vi "exam2.vi"() -> ()   [LabVIEW 2019]
uses:
  <vilib>/myRIO/Instrument Drivers/Onboard IO/DIO/typedefs/DIO Reference.ctl
  <vilib>/myRIO/Common/Instrument Driver Framework/Utilities/typedefs/myRIO Generic Hardware Reference.ctl
  <vilib>/myRIO/Common/Instrument Driver Framework/Utilities/typedefs/Hardware Version Enum.ctl
  <vilib>/myRIO/Common/Instrument Driver Framework/Utilities/typedefs/myRIO v1.0 Reference.ctl
  <vilib>/myRIO/Common/Instrument Driver Framework/Utilities/typedefs/Generic FPGA Reference.ctl
  <vilib>/myRIO/Common/Instrument Driver Framework/myRIO v1.0/DIO/typedefs/DIO Channels List.ctl
  <vilib>/myRIO/Common/Instrument Driver Framework/myRIO v1.0/DIO/typedefs/DIO Channels Enum.ctl
  <vilib>/userDefined/High Color/nirio_resource_hc.ctl
  <vilib>/userDefined/High Color/IMAQdx.ctl
  <vilib>/myRIO/Instrument Drivers/Onboard IO/PWM/typedefs/PWM Reference.ctl
  <vilib>/myRIO/Common/Instrument Driver Framework/myRIO v1.0/PWM/typedefs/PWM Channels Enum.ctl
  <vilib>/myRIO/Instrument Drivers/Onboard IO/PWM/typedefs/PWM Configuration.ctl
  <vilib>/myRIO/Common/Instrument Driver Framework/Utilities/vis/Is FPGA Ref Available.vi
  <vilib>/myRIO/Common/Instrument Driver Framework/myRIO v1.0/DIO/vis/myRIO v1.1 Open DIO.vi
  <vilib>/myRIO/Instrument Drivers/Onboard IO/DIO/vis/Write.vi
  <vilib>/myRIO/Common/Instrument Driver Framework/myRIO v1.0/PWM/vis/myRIO v1.1 Open PWM.vi
  <vilib>/myRIO/Common/Instrument Driver Framework/Utilities/vis/Validate Channels.vi
  <vilib>/myRIO/Common/Instrument Driver Framework/myRIO v1.0/DIO/vis/myRIO v1.0 Reserve DIO.vi
  <vilib>/myRIO/Common/Instrument Driver Framework/myRIO v1.0/PWM/vis/myRIO v1.0 Reserve PWM.vi
  <vilib>/myRIO/Common/Instrument Driver Framework/myRIO v1.0/PWM/vis/myRIO v1.0 Close PWM.vi
  <vilib>/myRIO/Common/Instrument Driver Framework/myRIO v1.0/Resource Manager/vis/myRIO v1.0 Reserve Channel List.vi
  <vilib>/myRIO/Common/Instrument Driver Framework/myRIO v1.0/DIO/vis/myRIO v1.0 Build MUX Configuration DIO.vi
  <vilib>/myRIO/Common/Instrument Driver Framework/myRIO v1.0/PWM/vis/myRIO v1.0 Build MUX Configuration PWM.vi
  <vilib>/myRIO/Common/Instrument Driver Framework/myRIO v1.0/PWM/vis/myRIO v1.0 Unreserve PWM.vi
  <vilib>/myRIO/Common/Instrument Driver Framework/myRIO v1.0/Resource Manager/vis/myRIO v1.0 Reserve Channel.vi
  <vilib>/myRIO/Common/Instrument Driver Framework/myRIO v1.0/Resource Manager/vis/myRIO v1.0 Unreserve Channel.vi
  <vilib>/myRIO/Common/Instrument Driver Framework/myRIO v1.0/Resource Manager/vis/myRIO v1.0 Create Configuration List.vi
  <vilib>/myRIO/Common/Instrument Driver Framework/myRIO v1.0/Resource Manager/vis/myRIO v1.0 Unreserve Channel List.vi
  <vilib>/myRIO/Common/Instrument Driver Framework/myRIO v1.0/Resource Manager/vis/myRIO v1.0 Build Mutex Name.vi
  <vilib>/Utility/VariantDataType/GetNumericInfo.vi
  <vilib>/Utility/error.llb/Error Cluster From Error Code.vi
  <vilib>/myRIO/Common/Instrument Driver Framework/myRIO v1.0/myRIO v1.1 Open.vi
  <vilib>/myRIO/Common/Instrument Driver Framework/Utilities/vis/IO Manager.vi
  <vilib>/myRIO/Common/Instrument Driver Framework/Utilities/vis/Configuration Manager.vi
  <vilib>/myRIO/Common/Instrument Driver Framework/myRIO v1.0/Resource Manager/vis/myRIO v1.0 Configure IO.vi
  <vilib>/myRIO/Common/Instrument Driver Framework/myRIO v1.0/myRIO v1.0 Close.vi
  <vilib>/myRIO/Common/Instrument Driver Framework/myRIO v1.0/PWM/vis/myRIO v1.0 Write PWM.vi
  <vilib>/myRIO/Common/Instrument Driver Framework/myRIO v1.0/PWM/vis/myRIO v1.0 Shutdown PWM.vi
  <vilib>/myRIO/Common/Instrument Driver Framework/myRIO v1.0/DIO/vis/myRIO v1.0 Write DIO.vi
  <vilib>/myRIO/Instrument Drivers/Onboard IO/PWM/vis/myRIO PWM Open.xnode
  <vilib>/myRIO/Express VI/Onboard IO/DO/DO Express VI.xnode
  <vilib>/myRIO/Instrument Drivers/Onboard IO/DIO/vis/myRIO DIO Open.xnode
  <vilib>/myRIO/Instrument Drivers/Onboard IO/PWM/PWM.lvlib
  <vilib>/vision/driver/NI_Vision_Acquisition_Software.lvlib
  <vilib>/myRIO/Instrument Drivers/Onboard IO/DIO/DIO.lvlib
panel:
  out "digital output":bool
  in  "reset":bool
  in  "LED stop":bool
  in  "webcam stop":bool
  out "picture":string
  out "Image":T1(plugin-control)
  in  "stop":bool
  in  "angle":dbl
  out "35«×":bool
  in  "Frequency [Hz]":dbl=1000.0
  out "duty cycle [%]":dbl
  in  "null offset":bool
  out "puls width [ms]":dbl
  out "offset":dbl
  in  "Channel Name":tag
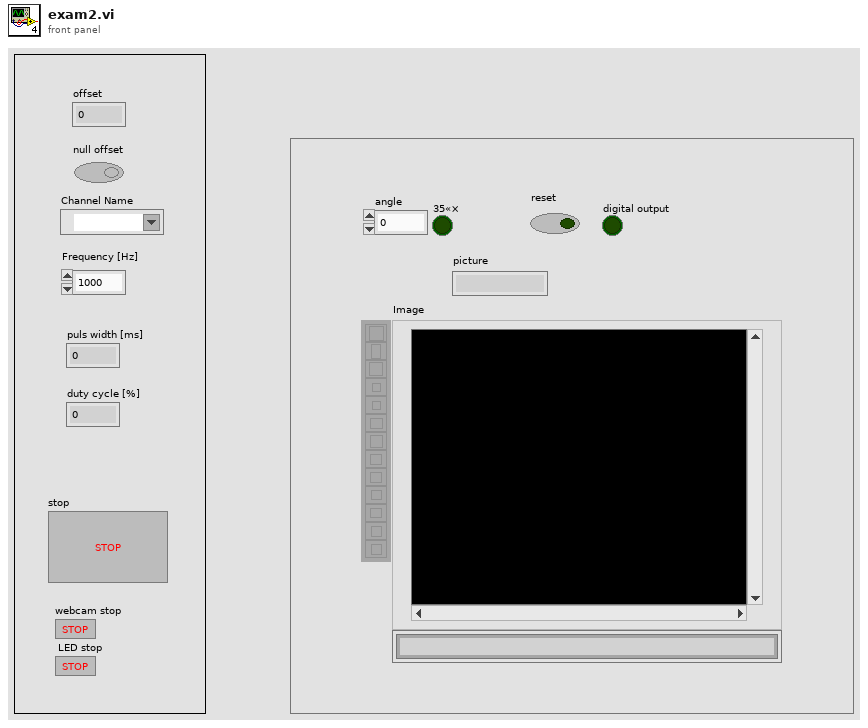
[diagram p1: front panel]
types:
  T1 = typedef "IMAQ Image.ctl" = refnum<image>
  T2 = typedef "PWM.lvlib/PWM Reference.ctl" = cluster{"myRIO Reference":T3, "PWM Channels Enum":T7, "PWM Configuration":T8}
  T3 = typedef "myRIO Generic Hardware Reference.ctl" = cluster{"myRIO Model":T4, "myRIO Hardware Reference":T5}
  T4 = typedef "Hardware Version Enum.ctl" = enum16{"Unknown", "myRIO-1900", "myRIO-1950", "roboRIO", "NI ELVIS RIO CM", "ELVIS III"}
  T5 = typedef "myRIO v1.0 Reference.ctl" = cluster{"Generic FPGA Reference":T6, "Allow multiple opens":bool}
  T6 = typedef "Generic FPGA Reference.ctl" = refnum<k20>
  T7 = typedef "PWM Channels Enum.ctl" = enum16{"Not Connected", "C/PWM0", "C/PWM1", "A/PWM0", "A/PWM1", "A/PWM2", "A/PWM3", "A/PWM4", "A/PWM5", "A/PWM6", "A/PWM7", "A/PWM8", "A/PWM9", "A/PWM10", "A/PWM11", "A/PWM12", "A/PWM13", "A/PWM14", "A/PWM15", "A/PWM16", "A/PWM17", "A/PWM18", "A/PWM19", "B/PWM0", "B/PWM1", "B/PWM2", "B/PWM3", "B/PWM4", "B/PWM5", "B/PWM6", "B/PWM7", "B/PWM8", "B/PWM9", "B/PWM10", "B/PWM11", "B/PWM12", "B/PWM13", "B/PWM14", "B/PWM15", "B/PWM16", "B/PWM17", "B/PWM18", "B/PWM19", "PWM/PWM0", "PWM/PWM1", "PWM/PWM2", "PWM/PWM3", "PWM/PWM4", "PWM/PWM5", "PWM/PWM6", "PWM/PWM7", "PWM/PWM8", "PWM/PWM9"}
  T8 = typedef "PWM.lvlib/PWM Configuration.ctl" = cluster{"Frequency":dbl, "Duty Cycle":dbl}
  T9 = typedef "IMAQdx.ctl" = refnum<k21>
  T10 = typedef "DIO.lvlib/DIO Reference.ctl" = cluster{"myRIO Reference":T3, "DIO Channels List":T11}
  T11 = typedef "DIO Channels List.ctl" = T12[]
  T12 = typedef "DIO Channels Enum.ctl" = enum16{"Not Connected", "C/DIO0", "C/DIO1", "C/DIO2", "C/DIO3", "C/DIO4", "C/DIO5", "C/DIO6", "C/DIO7", "A/DIO0", "A/DIO1", "A/DIO2", "A/DIO3", "A/DIO4", "A/DIO5", "A/DIO6", "A/DIO7", "A/DIO8", "A/DIO9", "A/DIO10", "A/DIO11", "A/DIO12", "A/DIO13", "A/DIO14", "A/DIO15", "A/DIO16", "A/DIO17", "A/DIO18", "A/DIO19", "B/DIO0", "B/DIO1", "B/DIO2", "B/DIO3", "B/DIO4", "B/DIO5", "B/DIO6", "B/DIO7", "B/DIO8", "B/DIO9", "B/DIO10", "B/DIO11", "B/DIO12", "B/DIO13", "B/DIO14", "B/DIO15", "B/DIO16", "B/DIO17", "B/DIO18", "B/DIO19", "LED0", "LED1", "LED2", "LED3", "Button0", "DIO/DIO0", "DIO/DIO1", "DIO/DIO2", "DIO/DIO3", "DIO/DIO4", "DIO/DIO5", "DIO/DIO6", "DIO/DIO7", "DIO/DIO8", "DIO/DIO9", "SPI/CS0", "SPI/CS1", "SPI/CS2", "SPI/CS3", "LED RADIO (Green)", "LED RADIO (Red)", "LED COMM (Green)", "LED COMM (Red)", "LED MODE (Green)", "LED MODE (Red)"}
  T13 = typedef "nirio_resource_hc.ctl" = tag
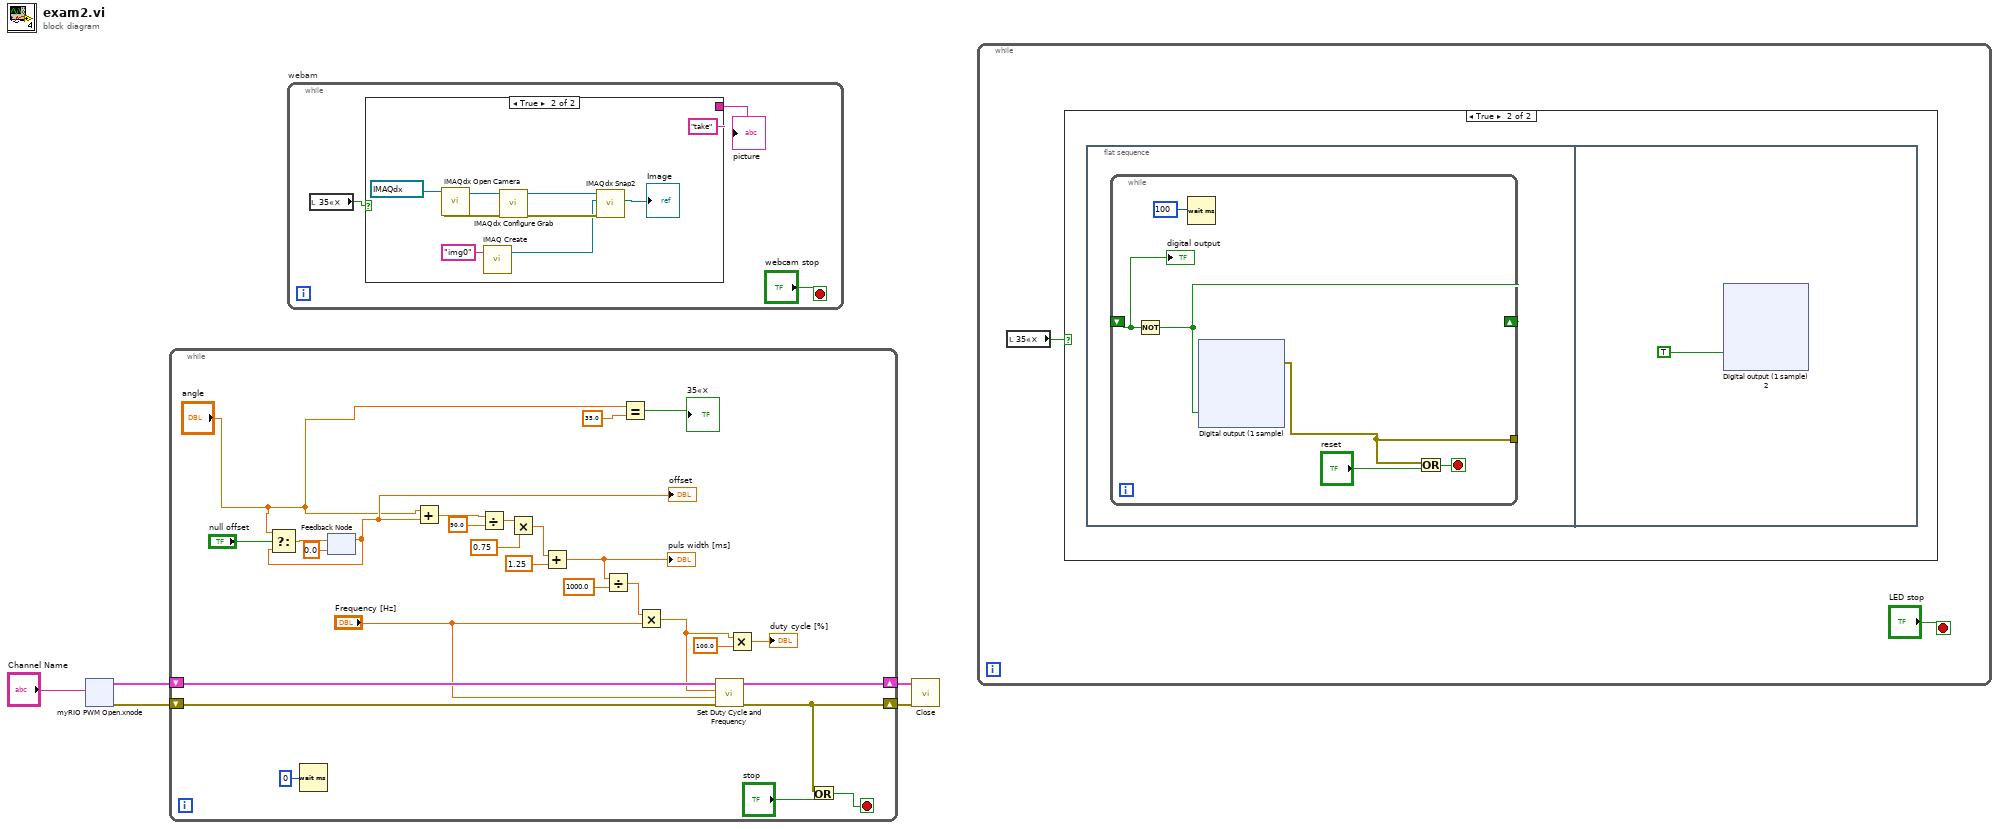
[diagram p0: block diagram]
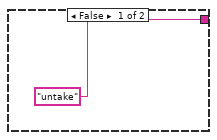
[diagram p3: hidden frame]
diagram:
  n1 = xnode "myRIO PWM Open.xnode"("Channel Name"="Channel Name") -> ("error out"=w4:errorcluster, "PWM Ref Out"=w3:T2)  [unwired: 2 in]
  n2 = while {
    shift-right: [w16] -> w2
    shift-left: w4 -> [w32]
    shift-right: [w30] -> w1
    shift-left: w3 -> [w31]
    stop <- w17 stop-if-true
    n3 = Wait (ms)(milliseconds to wait=u32 0) -> ()  [unwired: 1 out]
    n4 = feedback #1(0.0) -> (w14:dbl)
    "offset" <- w14
    n5 = Select(t="angle", s="null offset", f=w14) -> (s? t:f=w25:dbl)
    n6 = feedback-in #1(w25) -> ()
    n7 = Add(x="angle", y=w14) -> (x+y=w10:dbl)
    n8 = Divide(x=w10, y=90.0) -> (x/y=w13:dbl)
    n9 = Multiply(x=w13, y=0.75) -> (x*y=w12:dbl)
    n10 = Add(x=w12, y=1.25) -> (x+y=w20:dbl)
    "puls width [ms]" <- w20
    n11 = Divide(x=w20, y=1000.0) -> (x/y=w18:dbl)
    n12 = Equal?(x="angle", y=35.0) -> (x = y?=→"35«×":bool)
    n13 = Multiply(x=w18, y="Frequency [Hz]") -> (x*y=w27:dbl)
    n14 = call <vilib>:"Set Duty Cycle and Frequency.vi"("error in (no error)"=w32, "Frequency [Hz]"="Frequency [Hz]", "Duty Cycle"=w27, "PWM Ref In"=w31) -> ("error out"=w16:errorcluster, "PWM Ref Out"=w30:T2)  [unwired: 5 in]
    n15 = Multiply(x=w27, y=100.0) -> (x*y=→"duty cycle [%]":dbl)
    n16 = Or(x=w16, y="stop") -> (x .or. y?=w17:bool)
  }
  n17 = while "webam" {
    stop <- "webcam stop" stop-if-true
    n18 = local read "35«×"() -> (w33:bool)
    n19 = case "webcam snap" shown="True" w33 {
      tunnel: ["untake" "take"] -> w35
      frame False {
      }
      frame True {
        n20 = call <vilib>:"IMAQdx Open Camera.vi"("Session In"=T9 "cam1") -> ("error out"=w42:errorcluster, "Session Out"=w44:T9)  [unwired: 9 in]
        n21 = call "IMAQ Create"("Image Name"="img0") -> ("New Image"=w40:T1)  [unwired: 4 in, 1 out]
        n22 = call <vilib>:"IMAQdx Configure Grab.vi"("error in"=w42, "Session In"=w44) -> ("error out"=w41:errorcluster, "Session Out"=w43:T9)  [unwired: 8 in]
        n23 = call <vilib>:"IMAQdx Snap2.vi"("error in"=w41, "Image In"=w40, "Session In"=w43) -> ("Image Out"=→"Image":T1)  [unwired: 6 in, 2 out]
      }
    }
    "picture" <- w35
  }
  n24 = call <vilib>:"Close.vi"("error in (no error)"=w2, "PWM Ref In"=w1) -> ()  [unwired: 9 in, 1 out]
  n25 = while {
    stop <- "LED stop" stop-if-true
    n26 = local read "35«×"() -> (w46:bool)
    n27 = case shown="True" w46 {
      frame False {
      }
      frame True {
        n28 = flat-sequence {
          frame #0 {
            n29 = while {
              shift-right: [w49] -> _
              shift-left: _ -> [w51]
              tunnel: [w52] -> _
              stop <- w53 stop-if-true
              n30 = Not(x=w51) -> (.not. x?=w49:bool)
              n31 = Wait (ms)(milliseconds to wait=u32 100) -> ()  [unwired: 1 out]
              n32 = xnode "Digital output (1 sample)"("B/DIO0 (Pin 11)"=w49) -> ("error out"=w52:errorcluster)  [unwired: 1 in]
              n33 = Or(x=w52, y="reset") -> (x .or. y?=w53:bool)
              "digital output" <- w51
            }
          }
          frame #1 {
            n34 = xnode "Digital output (1 sample) 2"("B/DIO0 (Pin 11)"=TRUE) -> ()  [unwired: 1 in, 1 out]
          }
        }
      }
    }
  }
